vi "Moving average.vi"(9 "Reset":bool, 10 "data":dbl, 11 "Samples to average":i32) -> (1 "Array":dbl[](array[numeric]), 3 "Average":dbl)   [LabVIEW 2019, in "Turret.lvlib"]
uses:
  Classes/Turret/Turret.lvlib
  <vilib>/Analysis/baseanly.llb/Mean (DBL).vi
  <vilib>/Analysis/NI_AALBase.lvlib
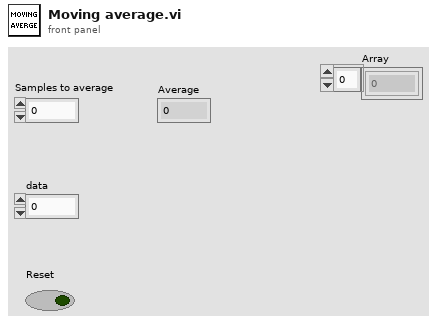
[diagram p1: front panel]
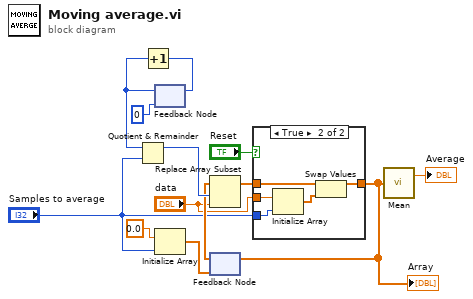
[diagram p0: block diagram]
diagram:
  n1 = feedback #1(0) -> (w10:i32)
  n2 = Quotient & Remainder(x=w10, y="Samples to average") -> (x-y*floor(x/y)=w8:i32)  [unwired: 1 out]
  n3 = Increment(x=w10) -> (x+1=w11:i32)
  n4 = feedback-in #1(w11) -> ()
  n5 = Initialize Array(0.0 ("element"), "Samples to average") -> (w6:dbl[])
  n6 = feedback #2(w6) -> (w7:dbl[])
  n7 = Replace Array Subset(array=w7, new element="data", index=w8) -> (w4:dbl[])
  n8 = case shown="True" "Reset" {
    tunnel: w4 -> [w14 w18]
    tunnel: [w14 w19] -> w3
    tunnel: "data" -> [_ w16]
    tunnel: "Samples to average" -> [_ w17]
    frame False {
    }
    frame True {
      n9 = Initialize Array(w16, w17) -> (w15:dbl[])
      n10 = Swap Values(12:w18, 14:w15) -> (1:w19:dbl[])  [unwired: 1 in, 1 out]
    }
  }
  "Array" <- w3
  n11 = feedback-in #2(w3) -> ()
  n12 = call-poly <vilib>:"Mean.vi"("X"=w3) -> ("mean"=→"Average":dbl)  [unwired: 1 out]
